vi "Compute IRF(X)PSED Plot.vi"(4 "Period T":dbl, 6 "Lifetime tau":dbl, 7 "Prefactor":dbl, 8 "error in (no error)":errorcluster, 9 "Decay X array":dbl[](array[numeric]), 10 "IRF Y Array":dbl[](array[numeric]), 11 "IRF X array":dbl[](array[numeric])) -> (0 "error out":errorcluster, 3 "IRF*PSED Plot":T1)   [LabVIEW 2021, in "Fits.lvlib"]
uses:
  Fits.lvlib
  Graphs/XY Graph/XY Plot Data.ctl
  Math/Math.lvlib
  Graphs/XY Graph/XY Graph Add-Ons.lvlib
  Utilities/Utilities.lvlib
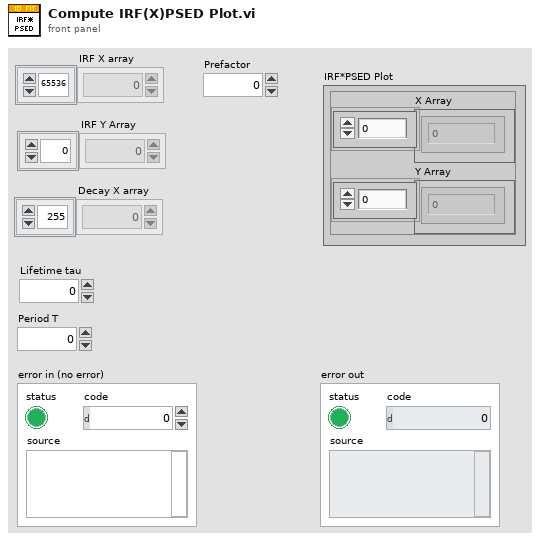
[diagram p1: front panel]
types:
  T1 = typedef "XY Graph Add-Ons.lvlib/XY Plot Data.ctl" = cluster{"X Array":dbl[], "Y Array":dbl[]}
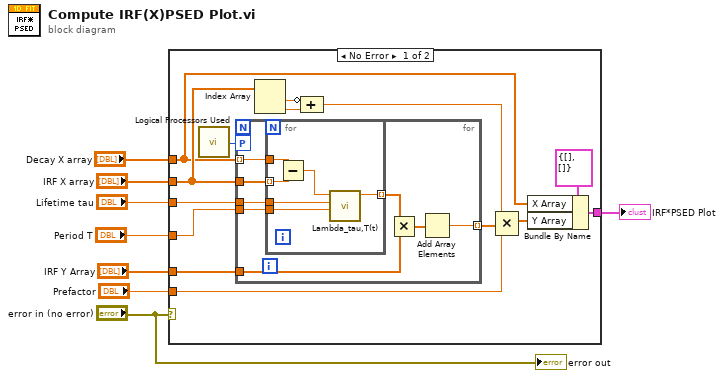
[diagram p0: block diagram]
diagram:
  n1 = case shown="No Error" "error in (no error)" {
    tunnel: "Lifetime tau" -> [w22 _]
    tunnel: "Period T" -> [w21 _]
    tunnel: "Decay X array" -> [w11 _]
    tunnel: "IRF Y Array" -> [w20 _]
    tunnel: "IRF X array" -> [w19 _]
    tunnel: [w13 _] -> w2
    tunnel: "Prefactor" -> [w10 _]
    frame No Error {
      n2 = call "Logical Processors Used.vi"() -> ("# Logical Processor Used"=w9:i32)  [unwired: 6 in]
      n3 = for {
        tunnel: w22 -> [w30]
        tunnel: w21 -> [w29]
        tunnel: w19 -> [w28]
        tunnel: w11 -> [w27] mode=indexing
        tunnel: w20 -> [w25]
        tunnel: [w23] -> w16 mode=indexing
        workers-P: w9 -> [_]
        n4 = for {
          tunnel: w30 -> [w36]
          tunnel: w29 -> [w35]
          tunnel: [w34] -> w26 mode=indexing
          tunnel: w28 -> [w32] mode=indexing
          tunnel: w27 -> [w33]
          n5 = Subtract(x=w33, y=w32) -> (x-y=w31:dbl)
          n6 = call "Lambda_tau,T(t).vi"("T"=w35, "tau"=w36, "t"=w31) -> ("Lambda_[tau,T](t)"=w34:dbl)  [unwired: 8 in]
        }
        n7 = Multiply(x=w26, y=w25) -> (x*y=w24:dbl[])
        n8 = Add Array Elements(numeric array=w24) -> (sum=w23:dbl)
      }
      n9 = Index Array(array=w19) -> (element #1=w17:dbl, element #2=w18:dbl)  [unwired: 2 in]
      n10 = Compound Arithmetic op=ADD(invert w17, w18) -> (w15:dbl)
      n11 = Compound Arithmetic op=MULTIPLY(w15, w16, w10) -> (w14:dbl[])
      n12 = Bundle By Name(cluster=T1 {"X Array"=[], "Y Array"=[]} ("IRF*PSED Plot"), "X Array"=w11, "Y Array"=w14) -> (w13:T1)
    }
    frame Error {
    }
  }
  "IRF*PSED Plot" <- w2
  "error out" <- "error in (no error)"
